vi "Get Object Pointer.vi"(11 "Data in":refnum<class "Data.lvclass">) -> (1 "Object Pointer":i64, 2 "Assigned object pointer?":bool, 3 "Data out":refnum<class "Data.lvclass">)   [LabVIEW 2015, in "MDSplus.lvlib" / "Data.lvclass"]
uses:
  <vilib>/MDSplus/Classes/Data_Class/Data.lvclass
  <vilib>/MDSplus/Classes/Data_Class/Data.lvclass/Data.ctl
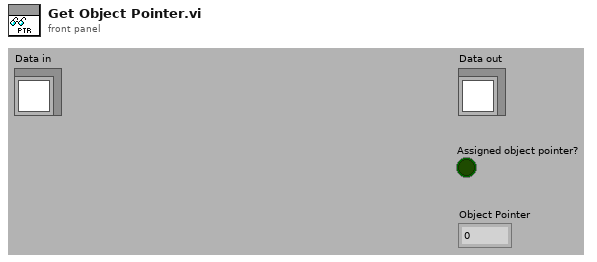
[diagram p1: front panel]
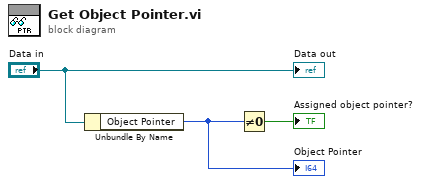
[diagram p0: block diagram]
diagram:
  n1 = Unbundle By Name("Data in") -> ("Object Pointer"=w1:i64)
  "Object Pointer" <- w1
  n2 = Not Equal To 0?(x=w1) -> (x != 0?=→"Assigned object pointer?":bool)
  "Data out" <- "Data in"
